vi "Periodic Tasks.vi"(11 "error out":errorcluster) -> ()   [LabVIEW 2011]
doc: "This VI runs in parallel to other tasks. It can contain as many user-defined periodic loops as you need. These can carry out PID or other sorts of timed response."
uses:
  PIDCluster.ctl
  <vilib>/Rock Robotics/WPI/Relay/WPI_RelayValue.ctl
  <vilib>/Rock Robotics/WPI/DriverStation/WPI_DriverStationRobotMode.ctl
  <vilib>/Rock Robotics/WPI/DriverStation/DriverStationLCD/WPI_DriverStationLCDLCDLine.ctl
  VisionData.vi
  <vilib>/Rock Robotics/WPI/Solenoid/Deprecated/WPI_SolenoidSetBool.vi
  <vilib>/addons/control/pid/pid.llb/PID (DBL).vi
  <vilib>/Rock Robotics/WPI/Compressor/WPI_CompressorGetSetRefNum.vi
  <vilib>/addons/control/pid/NI_PID_pid.lvlib
  <vilib>/Utility/file.llb/Read From Spreadsheet File (string).vi
  <vilib>/Utility/file.llb/Write To Spreadsheet File (string).vi
panel:
  in  "inner roller reverse time":dbl=0.5
  in  "visiondrive range":cluster{"output high":dbl, "output low":dbl}={"output high"=0.35, "output low"=-0.35}
  out "s? t:f":dbl
  out "Button 3":bool
  in  "visionDrive PID":T1={"proportional gain (Kc)"=2.0, "integral time (Ti, min)"=0.01, "derivative time (Td, min)"=0.0} {"derivative time (Td, min)" format="%.3f"; "integral time (Ti, min)" format="%.3f"; "proportional gain (Kc)" format="%.3f"}
  in  "upper limit":dbl=0.25
  in  "multiplier":dbl=-2.5
  out "most recent exe. time":u32
  out "extraneous times":u32[](array[numeric])
  out "left encoder":dbl
  in  "dedband":dbl=0.1 step=0.01
  in  "power constant":dbl=1.0
  out "output":dbl
  out "right encoder":dbl
  in  "lockdown pid gains":T1={"proportional gain (Kc)"=1.0, "integral time (Ti, min)"=0.01, "derivative time (Td, min)"=0.0} {"derivative time (Td, min)" format="%.3f"; "integral time (Ti, min)" format="%.3f"; "proportional gain (Kc)" format="%.3f"}
  in  "shift (overcome friction)":dbl=-0.22
  out "-1 to 1 CurrentCenter Value":dbl
  in  "PID gains":T2={"P"=0.005, "I"=0.003, "D"=0.0} {"D" format="%.3f"; "I" format="%.3f"; "P" format="%.3f"}
  out "iterations":i32
  in  "enable poops?":bool
  in  "RPM Deadband":dbl=20.0
  in  "ticks deadband":dbl=10.0
  in  "percent output (lockdown)":dbl=20.0
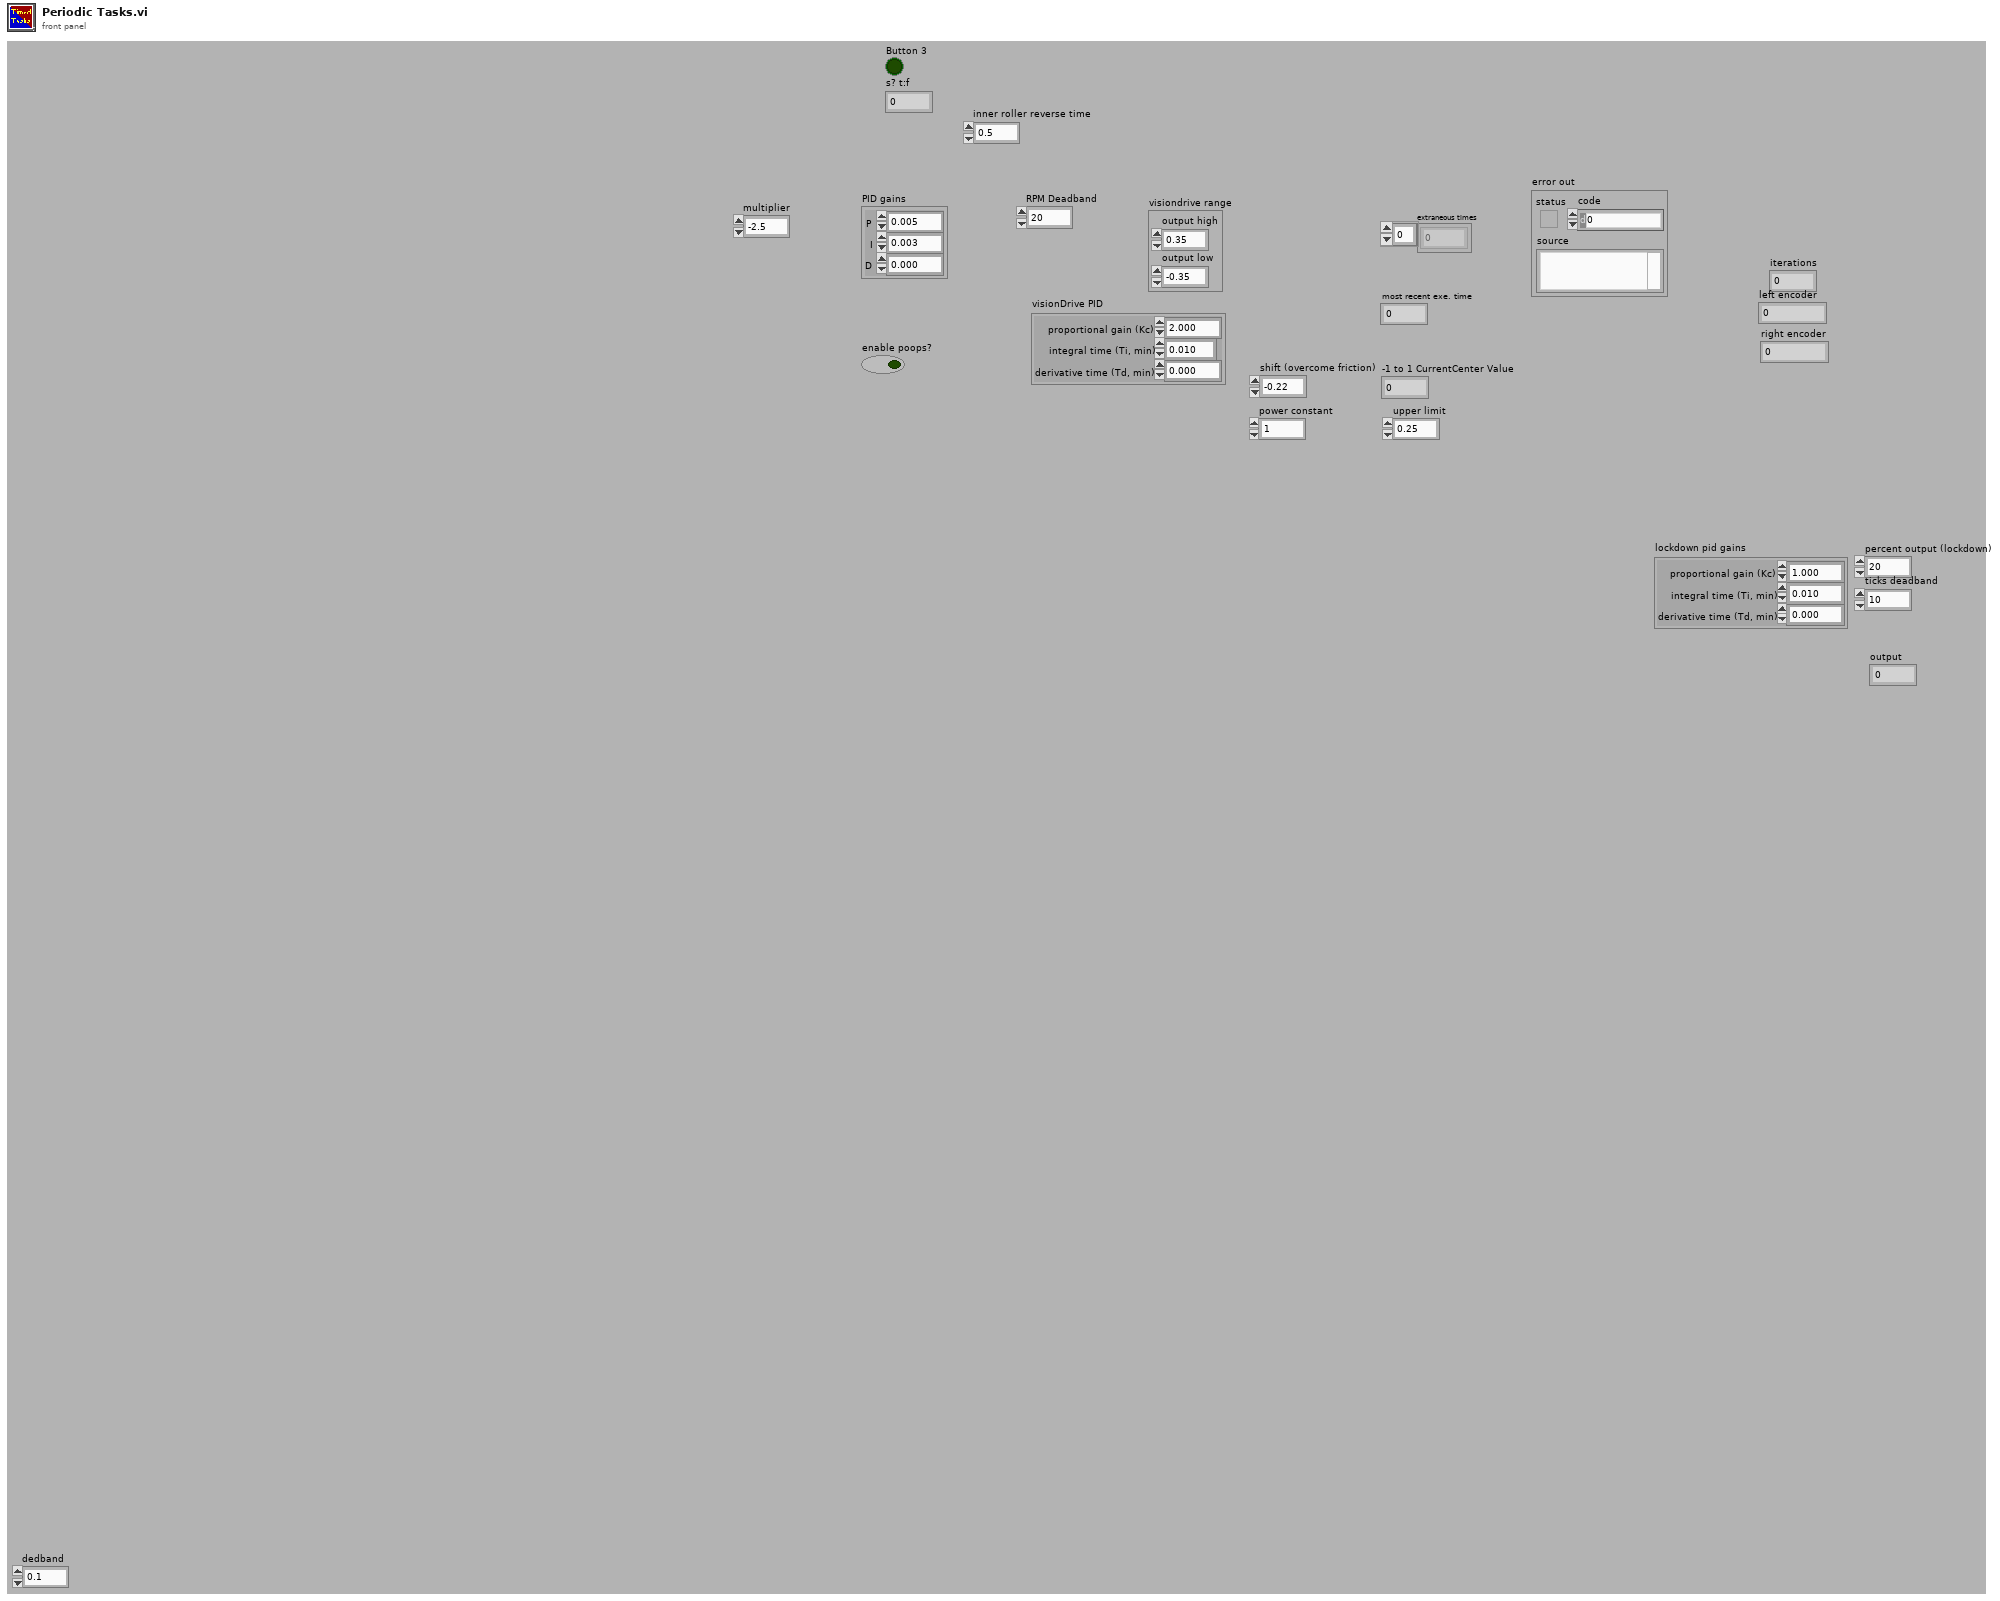
[diagram p1: front panel]
types:
  T1 = cluster{"proportional gain (Kc)":dbl, "integral time (Ti, min)":dbl, "derivative time (Td, min)":dbl}
  T2 = typedef "PIDCluster.ctl" = cluster{"P":dbl, "I":dbl, "D":dbl}
  T3 = typedef "WPI_MotorControlDeviceRef.ctl" = cluster{"DeviceStatus":errorcluster, "Type":enum16{"PWM", "CAN"}, "PWM":cluster{"Digital Module":T4, "PWM Channel":T5, "DeadBand":T6}, "CAN":cluster{"Device Number":u8, "Control Mode":T7, "Semaphore":T8, "Max Vout":dbl}, "Invert":bool, "TransformRef":T9, "InvTransformRef":T9}
  T4 = typedef "FPGA_TypedefDigitalModule.ctl" = enum16{"Digital Module 1", "Digital Module 2"}
  T5 = typedef "FPGA_DIOPWMChannel.ctl" = enum8{"PWM 1", "PWM 2", "PWM 3", "PWM 4", "PWM 5", "PWM 6", "PWM 7", "PWM 8", "PWM 9", "PWM 10", "Invalid"}
  T6 = typedef "WPI_PWMDeadband.ctl" = cluster{"Name":string, "maxPositivePwm":i32, "minPositivePwm":i32, "centerPwm":i32, "maxNegativePwm":i32, "minNegativePwm":i32, "angularRange":u16}
  T7 = typedef "WPI_CANJaguar_ControlMode.ctl" = enum8{"Percent VBus", "Current", "Speed", "Position", "Voltage"}
  T8 = typedef "Semaphore RefNum" = refnum<k1>
  T9 = typedef "WPI_PWMTransform_ConPane.ctl" = refnum<vi>
  T10 = typedef "WPI_SolenoidDevRef.ctl" = cluster{"DevStatus":errorcluster, "Solenoid Module":T11, "Forward Solenoid Channel":T12, "Reverse Solenoid Channel":T12}
  T11 = typedef "FPGA_TypedefSolenoidModule.ctl" = enum16{"Solenoid Module 1", "Solenoid Module 2"}
  T12 = typedef "WPI_SolenoidChannel.ctl" = enum8{"Solenoid 1", "Solenoid 2", "Solenoid 3", "Solenoid 4", "Solenoid 5", "Solenoid 6", "Solenoid 7", "Solenoid 8", "Invalid"}
  T13 = typedef "WPI_DigitalInputDevRef.ctl" = cluster{"DevStatus":errorcluster, "DIO Channel":T14, "Digital Module":T4}
  T14 = typedef "FPGA_DIOChannel.ctl" = enum8{"DIO 1", "DIO 2", "DIO 3", "DIO 4", "DIO 5", "DIO 6", "DIO 7", "DIO 8", "DIO 9", "DIO 10", "DIO 11", "DIO 12", "DIO 13", "DIO 14", "Invalid"}
  T15 = typedef "WPI_RelayDevRef.ctl" = cluster{"DevStatus":errorcluster, "Relay Channel":T16, "Digital Module":T4, "Relay Direction":T17}
  T16 = typedef "FPGA_DIORelayChannel.ctl" = enum8{"Relay 1", "Relay 2", "Relay 3", "Relay 4", "Relay 5", "Relay 6", "Relay 7", "Relay 8", "Invalid"}
  T17 = typedef "WPI_RelayDirection.ctl" = enum16{"Both directions", "Forward only", "Reverse only"}
  T18 = typedef "WPI_JoystickDevRef.ctl" = cluster{"Device":T19}
  T19 = typedef "WPI_JoystickDeviceEnum.ctl" = enum16{"USB 1", "USB 2", "USB 3", "USB 4", "Kinect 1", "Kinect 2"}
  T20 = typedef "WPI_EncoderDevRef.ctl" = cluster{"DevStatus":errorcluster, "EncoderIndex":T21, "CounterIndex":T22, "DistancePerCount":dbl, "Decoding Type":T23}
  T21 = typedef "FPGA_EncoderIdx.ctl" = enum8{"Enc 0", "Enc 1", "Enc 2", "Enc 3", "Invalid"}
  T22 = typedef "FPGA_CounterCtrSystemIndex.ctl" = enum8{"Ctr 0", "Ctr 1", "Ctr 2", "Ctr 3", "Ctr 4", "Ctr 5", "Ctr 6", "Ctr 7", "Invalid"}
  T23 = typedef "WPI_EncoderType.ctl" = enum16{"1x", "2x", "4x"}
  T24 = typedef "WPI_CounterDevRef.ctl" = cluster{"DevStatus":errorcluster, "CntIndex":T22}
  T25 = typedef "WPI_RelayValue.ctl" = enum16{"Off", "On", "Forward", "Reverse"}
  T26 = typedef "WPI_DriverStationRobotMode.ctl" = enum16{"Autonomous Disabled", "Autonomous Enabled", "Teleop Disabled", "Teleop Enabled", "Timeout", "Finish"}
  T27 = typedef "WPI_DriverStationLCDLCDLine.ctl" = enum16{"Main - Line 1", "User - Line 2", "User - Line 3", "User - Line 4", "User - Line 5", "User - Line 6"}
  T28 = typedef "WPI_JoystickButtonState.ctl" = cluster{"Button 1":bool, "Button 2":bool, "Button 3":bool, "Button 4":bool, "Button 5":bool, "Button 6":bool, "Button 7":bool, "Button 8":bool, "Button 9":bool, "Button 10":bool, "Button 11":bool, "Button 12":bool}
  T29 = cluster{"axis 1 (x)":dbl, "axis 2 (y)":dbl, "axis 3 (throttle)":dbl, "axis 4":dbl, "axis 5":dbl, "axis 6":dbl}
  T30 = cluster{"Position":cluster{"X":dbl, "Y":dbl}, "Distance (ft)":dbl, "NoTarget":bool, "Right":bool, "Center":bool, "Left":bool, "-1 to 1 CurrentCenter Value":dbl}
  T31 = typedef "WPI_CompressorDevRef.ctl" = cluster{"DevStatus":errorcluster, "DigitalInputDevRef":T13, "RelayDevRef":T15}
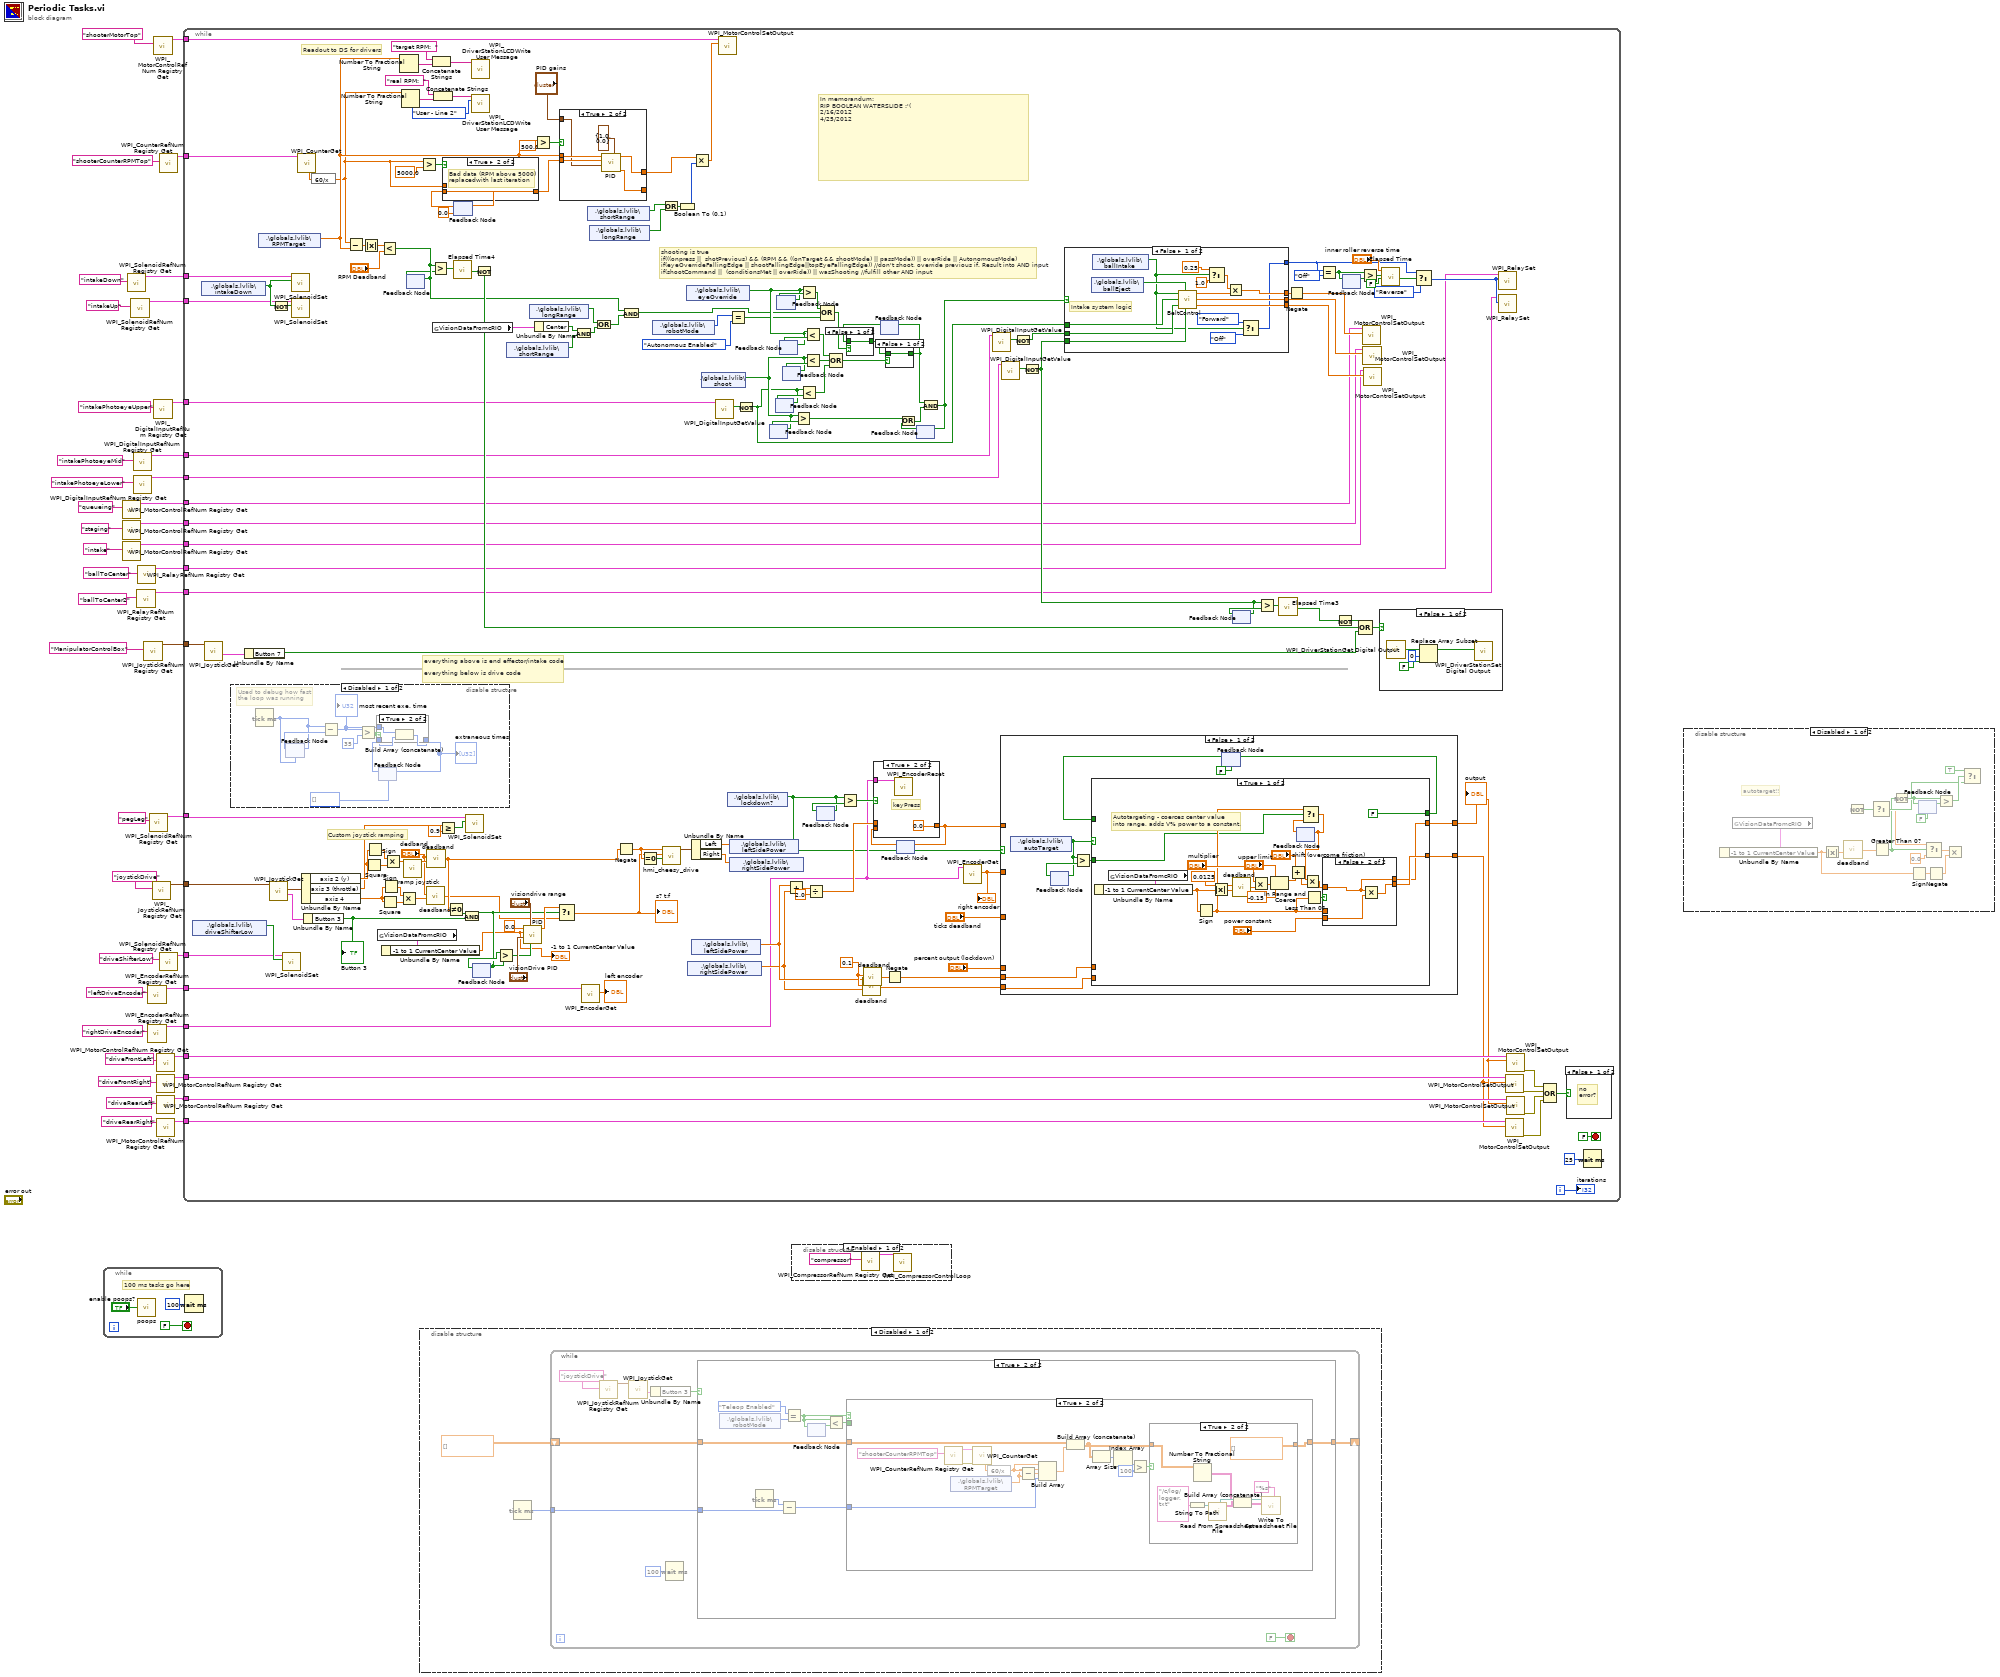
[diagram p0: block diagram]
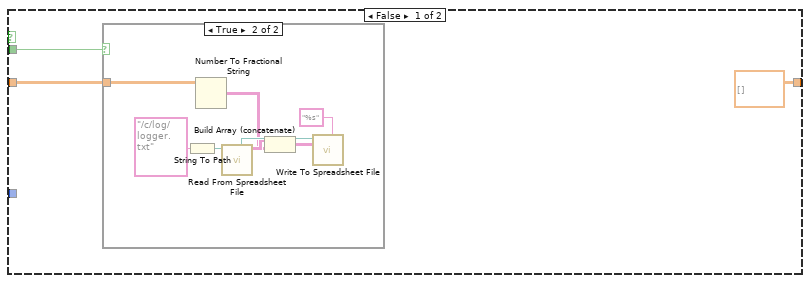
[diagram p4: hidden frame]
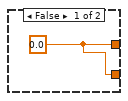
[diagram p11: hidden frame]
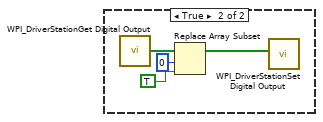
[diagram p12: hidden frame]
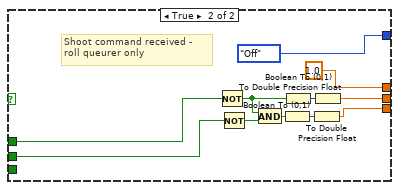
[diagram p14: hidden frame]
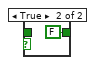
[diagram p15: hidden frame]
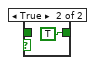
[diagram p16: hidden frame]
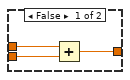
[diagram p17: hidden frame]
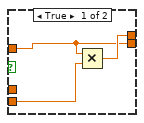
[diagram p18: hidden frame]
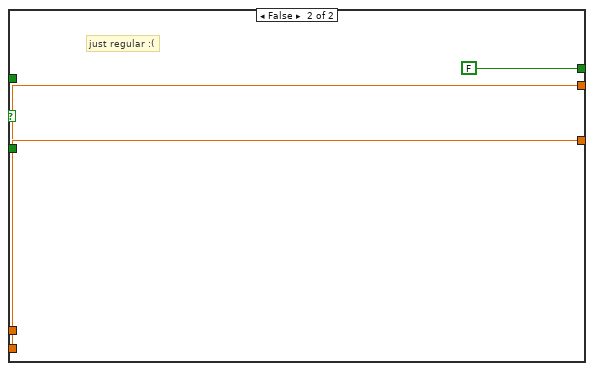
[diagram p19: hidden frame]
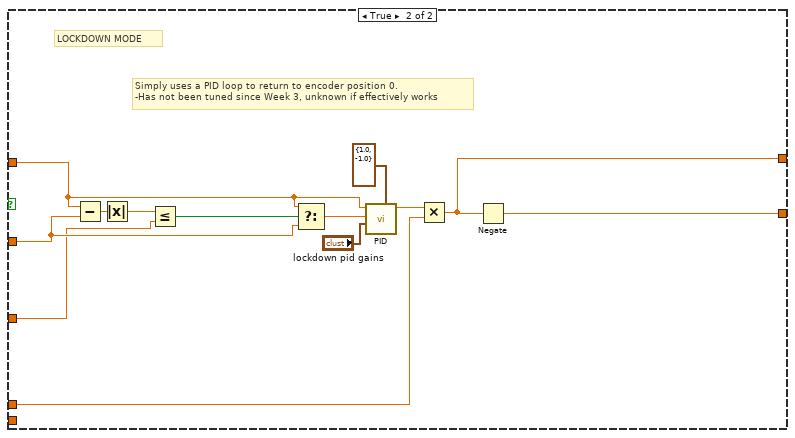
[diagram p20: hidden frame]
diagram:
  n1 = while {
    stop <- FALSE stop-if-true
    # "100 ms tasks go here"
    n2 = call "poops.vi"("enabled?"="enable poops?") -> ()  [unwired: 2 in]
    n3 = Wait (ms)(milliseconds to wait=u32 100) -> ()  [unwired: 1 out]
  }
  n4 = call <vilib>:"WPI_MotorControlRefNum Registry Get.vi"("refnum name"="queueing") -> ("MotorControlDevRef"=w31:T3)  [unwired: 9 in, 1 out]
  n5 = call <vilib>:"WPI_MotorControlRefNum Registry Get.vi"("refnum name"="staging") -> ("MotorControlDevRef"=w5:T3)  [unwired: 9 in, 1 out]
  n6 = call <vilib>:"WPI_MotorControlRefNum Registry Get.vi"("refnum name"="intake") -> ("MotorControlDevRef"=w30:T3)  [unwired: 9 in, 1 out]
  n7 = call <vilib>:"WPI_SolenoidRefNum Registry Get.vi"("refnum name"="intakeDown") -> ("SolenoidDevRef"=w38:T10)  [unwired: 9 in, 1 out]
  n8 = call <vilib>:"WPI_SolenoidRefNum Registry Get.vi"("refnum name"="intakeUp") -> ("SolenoidDevRef"=w37:T10)  [unwired: 9 in, 1 out]
  n9 = call <vilib>:"WPI_DigitalInputRefNum Registry Get.vi"("refnum name"="intakePhotoeyeMid") -> ("DigitalInputDevRef"=w7:T13)  [unwired: 9 in, 1 out]
  n10 = call <vilib>:"WPI_DigitalInputRefNum Registry Get.vi"("refnum name"="intakePhotoeyeLower") -> ("DigitalInputDevRef"=w6:T13)  [unwired: 9 in, 1 out]
  n11 = call <vilib>:"WPI_RelayRefNum Registry Get.vi"("refnum name"="ballToCenter2") -> ("RelayDevRef"=w1:T15)  [unwired: 9 in, 1 out]
  n12 = call <vilib>:"WPI_RelayRefNum Registry Get.vi"("refnum name"="ballToCenter") -> ("RelayDevRef"=w2:T15)  [unwired: 9 in, 1 out]
  n13 = call <vilib>:"WPI_JoystickRefNum Registry Get.vi"("refnum name"="ManipulatorControlBox") -> ("JoystickDevRef"=w43:T18)  [unwired: 1 in, 9 out]
  n14 = call <vilib>:"WPI_EncoderRefNum Registry Get.vi"("refnum name"="leftDriveEncoder") -> ("EncoderDevRef"=w21:T20)  [unwired: 9 in, 1 out]
  n15 = call <vilib>:"WPI_EncoderRefNum Registry Get.vi"("refnum name"="rightDriveEncoder") -> ("EncoderDevRef"=w20:T20)  [unwired: 9 in, 1 out]
  n16 = call <vilib>:"WPI_SolenoidRefNum Registry Get.vi"("refnum name"="pegLeg") -> ("SolenoidDevRef"=w10:T10)  [unwired: 9 in, 1 out]
  n17 = call <vilib>:"WPI_JoystickRefNum Registry Get.vi"("refnum name"="joystickDrive") -> ("JoystickDevRef"=w26:T18)  [unwired: 1 in, 9 out]
  n18 = call <vilib>:"WPI_MotorControlRefNum Registry Get.vi"("refnum name"="shooterMotorTop") -> ("MotorControlDevRef"=w35:T3)  [unwired: 9 in, 1 out]
  n19 = call <vilib>:"WPI_DigitalInputRefNum Registry Get.vi"("refnum name"="intakePhotoeyeUpper") -> ("DigitalInputDevRef"=w28:T13)  [unwired: 9 in, 1 out]
  n20 = call <vilib>:"WPI_MotorControlRefNum Registry Get.vi"("refnum name"="driveFrontRight") -> ("MotorControlDevRef"=w14:T3)  [unwired: 9 in, 1 out]
  n21 = call <vilib>:"WPI_MotorControlRefNum Registry Get.vi"("refnum name"="driveFrontLeft") -> ("MotorControlDevRef"=w15:T3)  [unwired: 9 in, 1 out]
  n22 = call <vilib>:"WPI_MotorControlRefNum Registry Get.vi"("refnum name"="driveRearLeft") -> ("MotorControlDevRef"=w13:T3)  [unwired: 9 in, 1 out]
  n23 = call <vilib>:"WPI_MotorControlRefNum Registry Get.vi"("refnum name"="driveRearRight") -> ("MotorControlDevRef"=w12:T3)  [unwired: 9 in, 1 out]
  n24 = call <vilib>:"WPI_CounterRefNum Registry Get.vi"("refnum name"="shooterCounterRPMTop") -> ("CounterDevRef"=w41:T24)  [unwired: 9 in, 1 out]
  n25 = call <vilib>:"WPI_SolenoidRefNum Registry Get.vi"("refnum name"="driveShifterLow") -> ("SolenoidDevRef"=w25:T10)  [unwired: 9 in, 1 out]
  n26 = while {
    tunnel: w43 -> [w107]
    tunnel: w41 -> [w96]
    tunnel: w38 -> [w93]
    tunnel: w37 -> [w94]
    tunnel: w35 -> [w95]
    tunnel: w31 -> [w50]
    tunnel: w5 -> [w51]
    tunnel: w30 -> [w52]
    tunnel: w28 -> [w91]
    tunnel: w26 -> [w90]
    tunnel: w25 -> [w89]
    tunnel: w21 -> [w88]
    tunnel: w20 -> [w58]
    tunnel: w15 -> [w87]
    tunnel: w14 -> [w86]
    tunnel: w13 -> [w85]
    tunnel: w12 -> [w84]
    tunnel: w10 -> [w83]
    tunnel: w7 -> [w60]
    tunnel: w6 -> [w59]
    tunnel: w2 -> [w54]
    tunnel: w1 -> [w53]
    i -> [w172]
    stop <- FALSE stop-if-true
    w189 = 0.1 ("tolerance")
    # "Custom joystick ramping"
    # "In memorandum:\nRIP BOOLEAN WATERSLIDE :'(\n2/16/2012\n4/25/2012"
    # "shooting is true\nif(((onpress ||  shotPrevious) && (RPM && ((onTarget && shootMode) || passMode)) || overRide || AutonomousMode)\nif(eyeOverrideFallingEdge || shootFallingEdge||topEyeFallingEdge)) //don't shoot, override previous if. Result into AND input\nif(shootCommand ||  (conditionsMet || overRide)) || wasShooting //fulfill other AND input"
    # "everything above is end effector/intake code\n\neverything below is drive code"
    # "Readout to DS for drivers"
    n27 = shared-variable ".\\globals.lvlib\\driveShifterLow"() -> (w190:bool)  [unwired: 1 in, 1 out]
    n28 = shared-variable ".\\globals.lvlib\\intakeDown"() -> (w187:bool)  [unwired: 1 in, 1 out]
    n29 = call <vilib>:"WPI_JoystickGet.vi"("JoystickDevRef"=w107) -> ("Buttons"=w74:T28)  [unwired: 1 in, 5 out]
    n30 = disable-structure shown="Disabled" {
      frame Disabled {
        # "Used to debug how fast\nthe loop was running"
        n31 = Tick Count (ms)() -> (millisecond timer value=w230:u32)
        n32 = feedback #1(w230) -> (w231:u32)
        n33 = feedback-in #1(w230) -> ()
        n34 = Subtract(x=w230, y=w231) -> (x-y=w224:u32)
        "most recent exe. time" <- w224
        n35 = Greater?(x=w224, y=u32 35) -> (0:w227:bool)
        n36 = feedback #2(i32[] []) -> (w225:u32[])
        n37 = case shown="True" w227 {
          tunnel: [w232 w234] -> w226
          tunnel: w225 -> [w232 w235]
          tunnel: w224 -> [_ w233]
          frame False {
          }
          frame True {
            n38 = Build Array (concatenate)(w233, w235) -> (w234:u32[])
          }
        }
        "extraneous times" <- w226
        n39 = feedback-in #2(w226) -> ()
      }
      frame Enabled {
      }
    }
    n40 = Unbundle By Name(w74) -> ("Button 7"=w104:bool)
    n41 = shared-variable ".\\globals.lvlib\\RPMTarget"() -> (w165:dbl)  [unwired: 1 in, 1 out]
    n42 = call <vilib>:"WPI_JoystickGet.vi"("JoystickDevRef"=w90) -> ("Buttons"=w152:T28, "Axes"=w210:T29)  [unwired: 1 in, 4 out]
    n43 = Not(x=w187) -> (.not. x?=w188:bool)
    n44 = call-poly <vilib>:"WPI_SolenoidSet.vi"("Value"=w190, "SolenoidDevRef"=w89) -> ()  [unwired: 8 in, 2 out]
    n45 = call-poly <vilib>:"WPI_SolenoidSet.vi"("Value"=w187, "SolenoidDevRef"=w93) -> ()  [unwired: 8 in, 2 out]
    n46 = call-poly <vilib>:"WPI_SolenoidSet.vi"("Value"=w188, "SolenoidDevRef"=w94) -> ()  [unwired: 8 in, 2 out]
    n47 = call <vilib>:"WPI_CounterGet.vi"("CounterDevRef in"=w96) -> ("Period (sec)"=w101:dbl)  [unwired: 5 in, 5 out]
    n48 = Unbundle By Name(w210) -> ("axis 2 (y)"=w133:dbl, "axis 3 (throttle)"=w127:dbl, "axis 4"=w116:dbl)
    n49 = Unbundle By Name(w152) -> ("Button 3"=w123:bool)
    "Button 3" <- w123
    n50 = expression code="60/x"(w101) -> (w161:dbl)
    n51 = Subtract(x=w161, y=w165) -> (x-y=w186:dbl)
    n52 = Absolute Value(x=w186) -> (abs(x)=w185:dbl)
    n53 = Square(x=w133) -> (x^2=w140:dbl)
    n54 = Sign(1:w133) -> (0:w139:dbl)
    n55 = global read "VisionData.vi" "VisionDataFromcRIO"() -> (w125:T30)
    n56 = Less?(x=w185, y="RPM Deadband") -> (x < y?=w100:bool)
    n57 = Square(x=w116) -> (x^2=w117:dbl)
    n58 = Unbundle By Name(w125) -> ("-1 to 1 CurrentCenter Value"=w82:dbl)
    "-1 to 1 CurrentCenter Value" <- w82
    n59 = Sign(1:w116) -> (0:w118:dbl)
    n60 = Multiply(x=w139, y=w140) -> (x*y=w132:dbl)
    n61 = Number To Fractional String(number=w165) -> (F-format string=w198:string)  [unwired: 3 in]
    n62 = Multiply(x=w118, y=w117) -> (x*y=w115:dbl)
    n63 = Number To Fractional String(number=w161) -> (F-format string=w195:string)  [unwired: 3 in]
    n64 = call "ramp joystick.vi"("joystick in"=w132) -> ("ramped joystick"=w121:dbl)  [unwired: 10 in]
    n65 = feedback #3() -> (w99:bool)  [unwired: 1 in]
    n66 = feedback-in #3(w100) -> ()
    n67 = Greater?(x=w161, y=5000.0) -> (0:w163:bool)
    n68 = call "deadband.vi"("tolerance"="dedband", "input"=w115) -> ("output"=w48:dbl)  [unwired: 5 in]
    n69 = call "deadband.vi"("tolerance"="dedband", "input"=w121) -> ("output"=w113:dbl)  [unwired: 5 in]
    n70 = Greater?(x=w100, y=w99) -> (0:w98:bool)
    n71 = Concatenate Strings("target RPM:  " ("string"), w198) -> (w194:string)
    n72 = global read "VisionData.vi" "VisionDataFromcRIO"() -> (w178:T30)
    n73 = Concatenate Strings("real RPM:  " ("string"), w195) -> (w193:string)
    n74 = Greater Or Equal?(x=w127, y=0.9) -> (x >= y?=w153:bool)
    n75 = Not Equal To 0?(x=w113) -> (x != 0?=w119:bool)
    n76 = call "Elapsed Time4"("Reset"=w98) -> ("Time has Elapsed"=w108:bool)  [unwired: 11 in, 7 out]
    n77 = feedback #4(0.0 ("Period (sec)")) -> (w162:dbl)
    n78 = case shown="True" w163 {
      tunnel: [w251 w252] -> w160
      tunnel: w161 -> [w251 _]
      tunnel: w162 -> [_ w252]
      frame False {
      }
      frame True {
        # "Bad data (RPM above 5000)\nreplacedwith last iteration"
      }
    }
    n79 = feedback-in #4(w160) -> ()
    n80 = And(x=w119, y=w123) -> (x .and. y?=w110:bool)
    n81 = call-poly <vilib>:"WPI_SolenoidSet.vi"("Value"=w153, "SolenoidDevRef"=w83) -> ()  [unwired: 8 in, 2 out]
    n82 = call <vilib>:"WPI_DriverStationLCDWrite User Message.vi"("line text"=w194) -> ()  [unwired: 14 in, 1 out]
    n83 = call <vilib>:"WPI_DriverStationLCDWrite User Message.vi"("line text"=w193, "line"=WPI_DriverStationLCDLCDLine."User - Line 2") -> ()  [unwired: 13 in, 1 out]
    n84 = feedback-in #5(w110) -> ()
    n85 = feedback #5() -> (w111:bool)  [unwired: 1 in]
    n86 = Not(x=w108) -> (.not. x?=w105:bool)
    n87 = Greater?(x=w111, y=w110) -> (0:w109:bool)
    n88 = shared-variable ".\\globals.lvlib\\shortRange"() -> (w176:bool)  [unwired: 1 in, 1 out]
    n89 = call-poly <vilib>:"PID.vi"("reinitialize? (F)"=w109, "output range"="visiondrive range", "PID gains"="visionDrive PID", "process variable"=w82, "setpoint"=0.0) -> ("output"=w114:dbl)  [unwired: 5 in, 1 out]
    n90 = shared-variable ".\\globals.lvlib\\longRange"() -> (w174:bool)  [unwired: 1 in, 1 out]
    n91 = Greater?(x=w165, y=500.0) -> (0:w218:bool)
    n92 = Unbundle By Name(w178) -> ("Center"=w177:bool)
    n93 = Select(t=w114, s=w110, f=w48) -> (s? t:f=w122:dbl)
    "s? t:f" <- w122
    n94 = case shown="True" w218 {
      tunnel: [w236 w241] -> w164
      tunnel: w160 -> [_ w240]
      tunnel: w165 -> [_ w239]
      tunnel: "PID gains" -> [_ w237]
      tunnel: [w236 w238] -> _
      frame False {
        w236 = 0.0 ("output")
      }
      frame True {
        n95 = call-poly <vilib>:"PID.vi"("output range"=cluster{"output high":dbl, "output low":dbl} {"output high"=1.0, "output low"=0.0}, "PID gains"=w237, "process variable"=w240, "setpoint"=w239) -> ("dt out (s)"=w238:dbl, "output"=w241:dbl)  [unwired: 6 in]
      }
    }
    n96 = And(x=w177, y=w176) -> (x .and. y?=w175:bool)
    n97 = call <vilib>:"WPI_EncoderGet.vi"("EncoderDevRef"=w88) -> ("Distance"=→"left encoder":dbl)  [unwired: 5 in, 5 out]
    n98 = shared-variable ".\\globals.lvlib\\shortRange"() -> (w166:bool)  [unwired: 1 in, 1 out]
    n99 = shared-variable ".\\globals.lvlib\\longRange"() -> (w191:bool)  [unwired: 1 in, 1 out]
    n100 = Or(x=w174, y=w175) -> (x .or. y?=w173:bool)
    n101 = Negate(x=w113) -> (-x=w134:dbl)
    n102 = And(x=w100, y=w173) -> (x .and. y?=w81:bool)
    n103 = Equal To 0?(x=w134) -> (x = 0?=w135:bool)
    n104 = shared-variable ".\\globals.lvlib\\robotMode"() -> (w171:u8)  [unwired: 1 in, 1 out]
    n105 = Or(x=w166, y=w191) -> (x .or. y?=w221:bool)
    n106 = call "hmi_cheesy_drive.vi"("Quick Turn"=w135, "Wheel"=w122, "Throttle"=w134) -> ("Drive Data"=w136:cluster{"Left":dbl, "Right":dbl})  [unwired: 8 in]
    n107 = Boolean To (0,1)(Boolean=w221) -> (0, 1=w220:i16)
    n108 = shared-variable ".\\globals.lvlib\\eyeOverride"() -> (w169:bool)  [unwired: 1 in, 1 out]
    n109 = shared-variable ".\\globals.lvlib\\rightSidePower"() -> (w141:dbl)  [unwired: 1 in, 1 out]
    n110 = Unbundle By Name(w136) -> ("Left"=w138:dbl, "Right"=w137:dbl)
    n111 = shared-variable ".\\globals.lvlib\\leftSidePower"() -> (w142:dbl)  [unwired: 1 in, 1 out]
    n112 = Multiply(x=w164, y=w220) -> (x*y=w102:dbl)
    n113 = shared-variable ".\\globals.lvlib\\shoot"() -> (w77:bool)  [unwired: 1 in, 1 out]
    n114 = call <vilib>:"WPI_DigitalInputGetValue.vi"("DigitalInputDevRef"=w91) -> ("Value"=w92:bool)  [unwired: 8 in, 2 out]
    n115 = call <vilib>:"WPI_MotorControlSetOutput.vi"("Output"=w102, "MotorControlDevRef"=w95) -> ()  [unwired: 8 in, 2 out]
    n116 = shared-variable ".\\globals.lvlib\\lockdown?"() -> (w57:bool)  [unwired: 1 in, 1 out]
    n117 = Equal?(x=w171, y=WPI_DriverStationRobotMode."Autonomous Enabled" ("Robot Mode")) -> (x = y?=w156:bool)
    n118 = shared-variable ".\\globals.lvlib\\leftSidePower"(w138) -> ()  [unwired: 1 in, 1 out]
    n119 = shared-variable ".\\globals.lvlib\\rightSidePower"(w137) -> ()  [unwired: 1 in, 1 out]
    n120 = Not(x=w92) -> (.not. x?=w61:bool)
    n121 = feedback #6() -> (w199:bool)  [unwired: 1 in]
    n122 = feedback-in #6(w77) -> ()
    n123 = feedback #7() -> (w207:bool)  [unwired: 1 in]
    n124 = feedback-in #7(w61) -> ()
    n125 = feedback #8() -> (w170:bool)  [unwired: 1 in]
    n126 = feedback-in #8(w169) -> ()
    n127 = feedback #9() -> (w203:bool)  [unwired: 1 in]
    n128 = feedback-in #9(w169) -> ()
    n129 = feedback #10() -> (w201:bool)  [unwired: 1 in]
    n130 = feedback-in #10(w77) -> ()
    n131 = Add(x=w142, y=w141) -> (x+y=w147:dbl)
    n132 = Greater?(x=w77, y=w199) -> (0:w209:bool)
    n133 = Greater?(x=w169, y=w170) -> (0:w158:bool)
    n134 = Less?(x=w61, y=w207) -> (x < y?=w204:bool)
    n135 = Less?(x=w169, y=w203) -> (x < y?=w79:bool)
    n136 = Less?(x=w77, y=w201) -> (x < y?=w200:bool)
    n137 = Divide(x=w147, y=2.0) -> (x/y=w145:dbl)
    n138 = feedback-in #11(w57) -> ()
    n139 = feedback #11() -> (w148:bool)  [unwired: 1 in]
    n140 = Compound Arithmetic op=OR(w158, w81, w156) -> (w155:bool)
    n141 = Compound Arithmetic op=OR(w79, w200, w204) -> (w205:bool)
    n142 = Greater?(x=w57, y=w148) -> (0:w149:bool)
    n143 = call "deadband.vi"("tolerance"=w189, "input"=w141) -> ("output"=w150:dbl)  [unwired: 5 in]
    n144 = call "deadband.vi"("tolerance"=w189, "input"=w142) -> ("output"=w183:dbl)  [unwired: 5 in]
    n145 = feedback #12() -> (w202:bool)  [unwired: 1 in]
    n146 = case shown="False" w155 {
      tunnel: [w281 TRUE] -> w206
      tunnel: w202 -> [w281 _]
      frame False {
      }
      frame True {
      }
    }
    n147 = case shown="False" w205 {
      tunnel: [w279 FALSE] -> w80
      tunnel: w206 -> [w279 _]
      frame False {
      }
      frame True {
      }
    }
    n148 = feedback-in #12(w80) -> ()
    n149 = Negate(x=w183) -> (-x=w151:dbl)
    n150 = feedback #13() -> (w144:dbl)  [unwired: 1 in]
    n151 = case shown="True" w149 {
      tunnel: w58 -> [_ w287]
      tunnel: w145 -> [w285 _]
      tunnel: [w283 0.0] -> w143
      tunnel: w144 -> [w284 _]
      frame False {
        n152 = Add(x=w285, y=w284) -> (x+y=w283:dbl)
      }
      frame True {
        # "keyPress"
        n153 = call <vilib>:"WPI_EncoderReset.vi"("EncoderDevRef"=w287) -> ()  [unwired: 9 in, 2 out]
      }
    }
    n154 = feedback-in #13(w143) -> ()
    n155 = feedback #14() -> (w168:bool)  [unwired: 1 in]
    n156 = Or(x=w209, y=w168) -> (x .or. y?=w78:bool)
    n157 = And(x=w80, y=w78) -> (x .and. y?=w167:bool)
    n158 = feedback-in #14(w167) -> ()
    n159 = call <vilib>:"WPI_EncoderGet.vi"("EncoderDevRef"=w58) -> ("Distance"=w211:dbl)  [unwired: 5 in, 5 out]
    "right encoder" <- w211
    n160 = call <vilib>:"WPI_DigitalInputGetValue.vi"("DigitalInputDevRef"=w60) -> ("Value"=w76:bool)  [unwired: 8 in, 2 out]
    n161 = case shown="False" w57 {
      tunnel: [w297 w335] -> w56
      tunnel: [w296 w340] -> w55
      tunnel: w151 -> [w288 _]
      tunnel: w150 -> [w289 _]
      tunnel: "percent output (lockdown)" -> [_ w338]
      tunnel: w211 -> [_ w337]
      tunnel: "ticks deadband" -> [_ w329]
      tunnel: w143 -> [_ w331]
      frame False {
        n162 = shared-variable ".\\globals.lvlib\\autoTarget"() -> (w291:bool)  [unwired: 1 in, 1 out]
        n163 = feedback-in #15(w291) -> ()
        n164 = feedback #15() -> (w292:bool)  [unwired: 1 in]
        n165 = Greater?(x=w291, y=w292) -> (0:w290:bool)
        n166 = feedback #16(FALSE) -> (w294:bool)
        n167 = case shown="True" w291 {
          tunnel: [w313 w326] -> w297
          tunnel: w288 -> [_ w326]
          tunnel: w289 -> [_ w327]
          tunnel: [w314 w327] -> w296
          tunnel: [FALSE FALSE] -> w293
          tunnel: w294 -> [_ _]
          tunnel: w290 -> [w298 _]
          frame True {
            # "Autotargeting - coerces center value \ninto range, adds V% power to a constant."
            n168 = global read "VisionData.vi" "VisionDataFromcRIO"() -> (w319:T30)
            n169 = Unbundle By Name(w319) -> ("-1 to 1 CurrentCenter Value"=w316:dbl)
            n170 = Sign(1:w316) -> (0:w306:dbl)
            n171 = Absolute Value(x=w316) -> (abs(x)=w318:dbl)
            n172 = call "deadband.vi"("tolerance"=0.0125, "input"=w318) -> ("output"=w310:dbl)  [unwired: 5 in]
            n173 = Multiply(x="multiplier", y=w310) -> (x*y=w304:dbl)
            n174 = In Range and Coerce(upper limit="upper limit", x=w304, lower limit=-0.15) -> (coerced(x)=w303:dbl)  [unwired: 1 out]
            n175 = Add(x="shift (overcome friction)", y=w303) -> (x+y=w300:dbl)
            n176 = feedback #17() -> (w311:dbl)  [unwired: 1 in]
            n177 = Select(t=w306, s=w298, f=w311) -> (s? t:f=w307:dbl)
            n178 = feedback-in #17(w307) -> ()
            n179 = Multiply(x=w307, y=w300) -> (x*y=w308:dbl)
            n180 = Less Than 0?(x=w306) -> (x < 0?=w315:bool)
            n181 = case shown="False" w315 {
              tunnel: w308 -> [w320 w323]
              tunnel: w306 -> [_ _]
              tunnel: [w320 w325] -> w314
              tunnel: [w322 w323] -> w313
              tunnel: "power constant" -> [w321 w324]
              frame True {
                n182 = Multiply(x=w320, y=w321) -> (x*y=w322:dbl)
              }
              frame False {
                n183 = Multiply(x=w323, y=w324) -> (x*y=w325:dbl)
              }
            }
          }
          frame False {
            # "just regular :("
          }
        }
        n184 = feedback-in #16(w293) -> ()
      }
      frame True {
        # "Simply uses a PID loop to return to encoder position 0.\n-Has not been tuned since Week 3, unknown if effectively works"
        # "LOCKDOWN MODE"
        n185 = Subtract(x=w331, y=w337) -> (x-y=w336:dbl)
        n186 = Absolute Value(x=w336) -> (abs(x)=w333:dbl)
        n187 = Less Or Equal?(x=w333, y=w329) -> (x <= y?=w334:bool)
        n188 = Select(t=w331, s=w334, f=w337) -> (s? t:f=w341:dbl)
        n189 = call-poly <vilib>:"PID.vi"("output range"=cluster{"output high":dbl, "output low":dbl} {"output high"=1.0, "output low"=-1.0}, "PID gains"="lockdown pid gains", "process variable"=w341, "setpoint"=w331) -> ("output"=w339:dbl)  [unwired: 6 in, 1 out]
        n190 = Multiply(x=w339, y=w338) -> (x*y=w335:dbl)
        n191 = Negate(x=w335) -> (-x=w340:dbl)
      }
    }
    "output" <- w56
    n192 = call <vilib>:"WPI_DigitalInputGetValue.vi"("DigitalInputDevRef"=w59) -> ("Value"=w75:bool)  [unwired: 8 in, 2 out]
    n193 = Not(x=w76) -> (.not. x?=w72:bool)
    n194 = Not(x=w75) -> (.not. x?=w73:bool)
    n195 = case shown="False" w167 {
      tunnel: [w258 1.0] -> w180
      tunnel: [w267 w277] -> w182
      tunnel: [w263 w271] -> w181
      tunnel: w61 -> [w266 w270]
      tunnel: w72 -> [w265 w269]
      tunnel: w73 -> [w264 _]
      tunnel: [w253 WPI_RelayValue."Off" ("RelayValue")] -> w63
      frame False {
        # "Intake system logic"
        n196 = shared-variable ".\\globals.lvlib\\ballEject"() -> (w262:bool)  [unwired: 1 in, 1 out]
        n197 = shared-variable ".\\globals.lvlib\\ballIntake"() -> (w254:bool)  [unwired: 1 in, 1 out]
        n198 = call "BeltControl.vi"("suck in"=w254, "roll out"=w262, "Top eye"=w266, "Middle eye"=w265, "Bottom eye"=w264) -> ("conveyerTop"=w261:dbl, "conveyerMiddle"=w267:dbl, "conveyerBottom"=w263:dbl)
        n199 = Select(t=0.25, s=w254, f=1.0) -> (s? t:f=w259:dbl)
        n200 = Multiply(x=w259, y=w261) -> (x*y=w258:dbl)
        n201 = Select(t=WPI_RelayValue."Forward" ("RelayValue"), s=w254, f=WPI_RelayValue."Off" ("RelayValue")) -> (s? t:f=w253:T25)
      }
      frame True {
        # "Shoot command received - \nroll queurer only"
        n202 = Not(x=w270) -> (.not. x?=w275:bool)
        n203 = Not(x=w269) -> (.not. x?=w274:bool)
        n204 = And(x=w275, y=w274) -> (x .and. y?=w272:bool)
        n205 = Boolean To (0,1)(Boolean=w272) -> (0, 1=w273:i16)
        n206 = Boolean To (0,1)(Boolean=w275) -> (0, 1=w276:i16)
        n207 = To Double Precision Float(number=w273) -> (double precision float=w271:dbl)
        n208 = To Double Precision Float(number=w276) -> (double precision float=w277:dbl)
      }
    }
    n209 = feedback #18() -> (w131:bool)  [unwired: 1 in]
    n210 = feedback-in #18(w73) -> ()
    n211 = Greater?(x=w73, y=w131) -> (0:w130:bool)
    n212 = call "Elapsed Time3"("Reset"=w130) -> ("Time has Elapsed"=w129:bool)  [unwired: 11 in, 7 out]
    n213 = Negate(x=w180) -> (-x=w179:dbl)
    n214 = Equal?(x=w63, y=WPI_RelayValue."Off") -> (x = y?=w65:bool)
    n215 = Not(x=w129) -> (.not. x?=w106:bool)
    n216 = feedback #19() -> (w66:bool)  [unwired: 1 in]
    n217 = feedback-in #19(w65) -> ()
    n218 = Compound Arithmetic op=OR(w106, w105, w104) -> (w103:bool)
    n219 = Greater?(x=w65, y=w66) -> (0:w67:bool)
    n220 = call <vilib>:"WPI_MotorControlSetOutput.vi"("Output"=w179, "MotorControlDevRef"=w50) -> ()  [unwired: 8 in, 2 out]
    n221 = call <vilib>:"WPI_MotorControlSetOutput.vi"("Output"=w182, "MotorControlDevRef"=w51) -> ()  [unwired: 8 in, 2 out]
    n222 = call <vilib>:"WPI_MotorControlSetOutput.vi"("Output"=w181, "MotorControlDevRef"=w52) -> ()  [unwired: 8 in, 2 out]
    n223 = case shown="False" w103 {
      frame False {
        n224 = call <vilib>:"WPI_DriverStationGet Digital Output.vi"() -> ("Driver Station Digital Output (1-8)"=w246:bool[])  [unwired: 10 in, 1 out]
        n225 = Replace Array Subset(array=w246, new element=FALSE ("new element/subarray"), index=0) -> (w243:bool[])
        n226 = call <vilib>:"WPI_DriverStationSet Digital Output.vi"("Driver Station Digital Output (1-8)"=w243) -> ()  [unwired: 10 in, 1 out]
      }
      frame True {
        n227 = call <vilib>:"WPI_DriverStationGet Digital Output.vi"() -> ("Driver Station Digital Output (1-8)"=w250:bool[])  [unwired: 10 in, 1 out]
        n228 = Replace Array Subset(array=w250, new element=TRUE ("new element/subarray"), index=0) -> (w247:bool[])
        n229 = call <vilib>:"WPI_DriverStationSet Digital Output.vi"("Driver Station Digital Output (1-8)"=w247) -> ()  [unwired: 10 in, 1 out]
      }
    }
    n230 = call "Elapsed Time"("Time Target (s)"="inner roller reverse time", "Reset"=w67, "Auto Reset"=FALSE) -> ("Time has Elapsed"=w68:bool)  [unwired: 9 in, 7 out]
    n231 = Select(t=w63, s=w68, f=WPI_RelayValue."Reverse") -> (s? t:f=w62:T25)
    n232 = call <vilib>:"WPI_RelaySet.vi"("RelayValue"=w62, "RelayDevRef"=w54) -> ()  [unwired: 8 in, 2 out]
    n233 = call <vilib>:"WPI_RelaySet.vi"("RelayValue"=w62, "RelayDevRef"=w53) -> ()  [unwired: 8 in, 2 out]
    n234 = call <vilib>:"WPI_MotorControlSetOutput.vi"("Output"=w55, "MotorControlDevRef"=w86) -> ("error out"=w216:errorcluster)  [unwired: 8 in, 1 out]
    n235 = call <vilib>:"WPI_MotorControlSetOutput.vi"("Output"=w55, "MotorControlDevRef"=w84) -> ("error out"=w214:errorcluster)  [unwired: 8 in, 1 out]
    n236 = call <vilib>:"WPI_MotorControlSetOutput.vi"("Output"=w56, "MotorControlDevRef"=w87) -> ("error out"=w217:errorcluster)  [unwired: 8 in, 1 out]
    n237 = call <vilib>:"WPI_MotorControlSetOutput.vi"("Output"=w56, "MotorControlDevRef"=w85) -> ("error out"=w215:errorcluster)  [unwired: 8 in, 1 out]
    n238 = Compound Arithmetic op=OR(w217, w216, w215, w214) -> (w213:bool)
    n239 = case shown="False" w213 {
      frame False {
        # "no error?"
      }
      frame True {
        # "Error simply dismissed"
      }
    }
    n240 = Wait (ms)(milliseconds to wait=u32 25) -> ()  [unwired: 1 out]
    "iterations" <- w172
  }
  n241 = disable-structure shown="Disabled" {
    frame Disabled {
      n242 = Tick Count (ms)() -> (millisecond timer value=w343:u32)
      n243 = while {
        shift-right: [w351] -> _
        shift-left: dbl[][] [] -> [w352]
        tunnel: w343 -> [w350]
        stop <- FALSE stop-if-true
        n244 = call <vilib>:"WPI_JoystickRefNum Registry Get.vi"("refnum name"="joystickDrive") -> ("JoystickDevRef"=w347:T18)  [unwired: 1 in, 9 out]
        n245 = call <vilib>:"WPI_JoystickGet.vi"("JoystickDevRef"=w347) -> ("Buttons"=w346:T28)  [unwired: 1 in, 5 out]
        n246 = Unbundle By Name(w346) -> ("Button 3"=w345:bool)
        n247 = Wait (ms)(milliseconds to wait=u32 100) -> ()  [unwired: 1 out]
        n248 = case shown="True" w345 {
          tunnel: w352 -> [w353 w363]
          tunnel: [w353 w362] -> w351
          tunnel: w350 -> [_ w360]
          frame False {
          }
          frame True {
            n249 = shared-variable ".\\globals.lvlib\\robotMode"() -> (w358:u8)  [unwired: 1 in, 1 out]
            n250 = Tick Count (ms)() -> (millisecond timer value=w361:u32)
            n251 = Subtract(x=w361, y=w360) -> (x-y=w359:u32)
            n252 = Equal?(x=WPI_DriverStationRobotMode."Teleop Enabled" ("Robot Mode"), y=w358) -> (x = y?=w356:bool)
            n253 = feedback #20() -> (w355:bool)  [unwired: 1 in]
            n254 = feedback-in #20(w356) -> ()
            n255 = Less?(x=w356, y=w355) -> (x < y?=w354:bool)
            n256 = case shown="True" w356 {
              tunnel: w363 -> [w365 w383]
              tunnel: [dbl[][] [] w377] -> w362
              tunnel: w359 -> [_ w376]
              tunnel: w354 -> [w364 _]
              frame False {
                n257 = case shown="True" w364 {
                  tunnel: w365 -> [_ w367]
                  frame False {
                  }
                  frame True {
                    n258 = String To Path(string="/c/log/logger.txt") -> (path=w373:path)
                    n259 = Number To Fractional String(number=w367) -> (F-format string=w369:string[][])  [unwired: 3 in]
                    n260 = call-poly <vilib>:"Read From Spreadsheet File.vi"("file path (dialog if empty)"=w373) -> ("all rows"=w370:string[][], "new file path (Not A Path if cancelled)"=w372:path)  [unwired: 6 in, 3 out]
                    n261 = Build Array (concatenate)(w370, w369) -> (w368:string[][])
                    n262 = call-poly <vilib>:"Write To Spreadsheet File.vi"("format (%s)"="%s" ("format (%.3f)"), "2D data"=w368, "file path (dialog if empty)"=w372) -> ()  [unwired: 5 in, 1 out]
                  }
                }
              }
              frame True {
                n263 = call <vilib>:"WPI_CounterRefNum Registry Get.vi"("refnum name"="shooterCounterRPMTop") -> ("error out"=w390:errorcluster, "CounterDevRef"=w388:T24)  [unwired: 9 in]
                n264 = shared-variable ".\\globals.lvlib\\RPMTarget"() -> (w385:dbl)  [unwired: 1 in, 1 out]
                n265 = call <vilib>:"WPI_CounterGet.vi"("error in (no error)"=w390, "CounterDevRef in"=w388) -> ("Period (sec)"=w389:dbl)  [unwired: 4 in, 5 out]
                n266 = expression code="60/x"(w389) -> (w386:dbl)
                n267 = Subtract(x=w386, y=w385) -> (x-y=w384:dbl)
                n268 = Build Array(w386, w385, w384, w376) -> (w382:dbl[])
                n269 = Build Array (concatenate)(w383, w382) -> (w380:dbl[][])
                n270 = Array Size(array=w380) -> (size(s)=w381:i32[])
                n271 = Index Array(array=w381) -> (element=w378:i32)  [unwired: 1 in]
                n272 = Greater?(x=w378, y=100) -> (0:w379:bool)
                n273 = case shown="True" w379 {
                  tunnel: w380 -> [w391 w395]
                  tunnel: [w391 dbl[][] []] -> w377
                  frame False {
                  }
                  frame True {
                    n274 = String To Path(string="/c/log/logger.txt") -> (path=w398:path)
                    n275 = Number To Fractional String(number=w395) -> (F-format string=w393:string[][])  [unwired: 3 in]
                    n276 = call-poly <vilib>:"Read From Spreadsheet File.vi"("file path (dialog if empty)"=w398) -> ("all rows"=w394:string[][], "new file path (Not A Path if cancelled)"=w397:path)  [unwired: 6 in, 3 out]
                    n277 = Build Array (concatenate)(w394, w393) -> (w392:string[][])
                    n278 = call-poly <vilib>:"Write To Spreadsheet File.vi"("format (%s)"="%s" ("format (%.3f)"), "2D data"=w392, "file path (dialog if empty)"=w397) -> ()  [unwired: 5 in, 1 out]
                  }
                }
              }
            }
          }
        }
      }
    }
    frame Enabled {
    }
  }
  n279 = disable-structure shown="Enabled" {
    frame Enabled {
      n280 = call <vilib>:"WPI_CompressorRefNum Registry Get.vi"("refnum name"="compressor") -> ("CompressorDevRef"=w402:T31)  [unwired: 9 in, 1 out]
      n281 = call <vilib>:"WPI_CompressorControlLoop.vi"("CompressorDevRef"=w402) -> ()  [unwired: 11 in]
    }
    frame Disabled {
    }
  }
  n282 = disable-structure shown="Disabled" {
    frame Disabled {
      # "autotarget!!"
      n283 = global read "VisionData.vi" "VisionDataFromcRIO"() -> (w419:T30)
      n284 = Unbundle By Name(w419) -> ("-1 to 1 CurrentCenter Value"=w416:dbl)
      n285 = Absolute Value(x=w416) -> (abs(x)=w412:dbl)
      n286 = call "deadband.vi"("input"=w412) -> ("output"=w415:dbl)  [unwired: 6 in]
      n287 = Greater Than 0?(x=w415) -> (x > 0?=w405:bool)
      n288 = Not(x=w405) -> (.not. x?=w410:bool)
      n289 = Sign(1:w416) -> (0:w418:dbl)
      n290 = feedback #21(FALSE) -> (w409:bool)
      n291 = feedback-in #21(w410) -> ()
      n292 = Negate(x=w418) -> (-x=w417:dbl)
      n293 = Greater?(x=w410, y=w409) -> (0:w408:bool)
      n294 = Select(t=TRUE, s=w408) -> (f=w406:bool)  [unwired: 1 out]
      n295 = Not(x=w406) -> (.not. x?=w404:bool)
      n296 = Select(s=w404) -> (s? t:f=w403:dbl)  [unwired: 2 in]
      n297 = Select(t=w403, s=w405, f=0.0) -> (s? t:f=w414:dbl)
      n298 = Multiply(x=w414, y=w417) -> ()  [unwired: 1 out]
    }
    frame Enabled {
    }
  }
